vi "Get Plugin Directory Path.vi"() -> (2 "Plugin map":map{string, path}(c390), 3 "Plugin Directory":path)   [LabVIEW 2020]
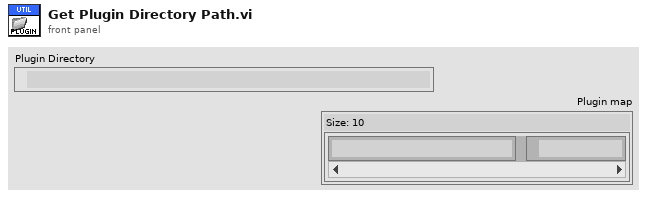
[diagram p1: front panel]
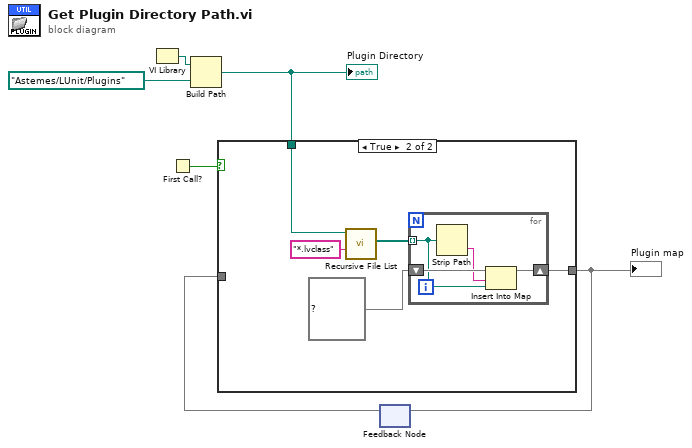
[diagram p0: block diagram]
diagram:
  n1 = VI Library() -> (path=w6:path)
  n2 = First Call?() -> (First Call?: T/F=w2:bool)
  n3 = Build Path(base path=w6, name or relative path=path "Astemes/LUnit/Plugins") -> (appended path=w4:path)
  "Plugin Directory" <- w4
  n4 = feedback #1() -> (w1:map{string, path})  [unwired: 1 in]
  n5 = case shown="True" w2 {
    tunnel: w4 -> [_ w9]
    tunnel: [w7 w8] -> w3
    tunnel: w1 -> [w7 _]
    frame False {
    }
    frame True {
      n6 = call <vilib>:"Recursive File List.vi"("pattern"="*.lvclass", "Folder Path"=w9) -> ("All Files in Dir"=w10:path[])  [unwired: 5 in, 4 out]
      n7 = for {
        shift-right: [w15] -> w8
        shift-left: map{string, path} {} ("map") -> [w16]
        tunnel: w10 -> [w13] mode=indexing
        n8 = Strip Path(path=w13) -> (name=w14:string)  [unwired: 1 out]
        n9 = Insert Into Map(map in=w16, key=w14, value=w13) -> (map out=w15:map{string, path})  [unwired: 2 out]
      }
    }
  }
  "Plugin map" <- w3
  n10 = feedback-in #1(w3) -> ()
